vi "Navigate and Wait.vi"(7 "html Source (URL)":bool, 8 "Error In":errorcluster, 9 "Timeout (Inf)":i32=-1, 10 "Source":string, 11 "WebView in":refnum<class "WebView.lvclass">) -> (0 "Error Out":errorcluster, 2 "Timed Out":bool, 3 "WebView out":refnum<class "WebView.lvclass">)   [LabVIEW 2020, in "WebView.lvclass"]
uses:
  WebView.lvclass
  <vilib>/sklein/WebView2/Libs/Microsoft.Web.WebView2.Core.dll
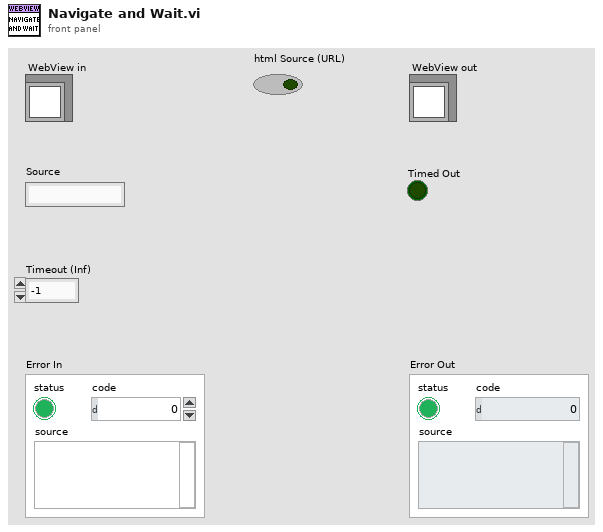
[diagram p1: front panel]
types:
  T1 = typedef "WebView.lvclass/Events--cluster.ctl" = cluster{"Navigation Complete Event":refnum<user-event>, "Source Changed Event":refnum<user-event>, "Document Title Changed Event":refnum<user-event>, "Status Bar Text Changed":refnum<user-event>, "Web Message Received":refnum<user-event>, "Window Close Requested":refnum<user-event>, "DOM Loaded":refnum<user-event>, "Navigation Started Event":refnum<user-event>}
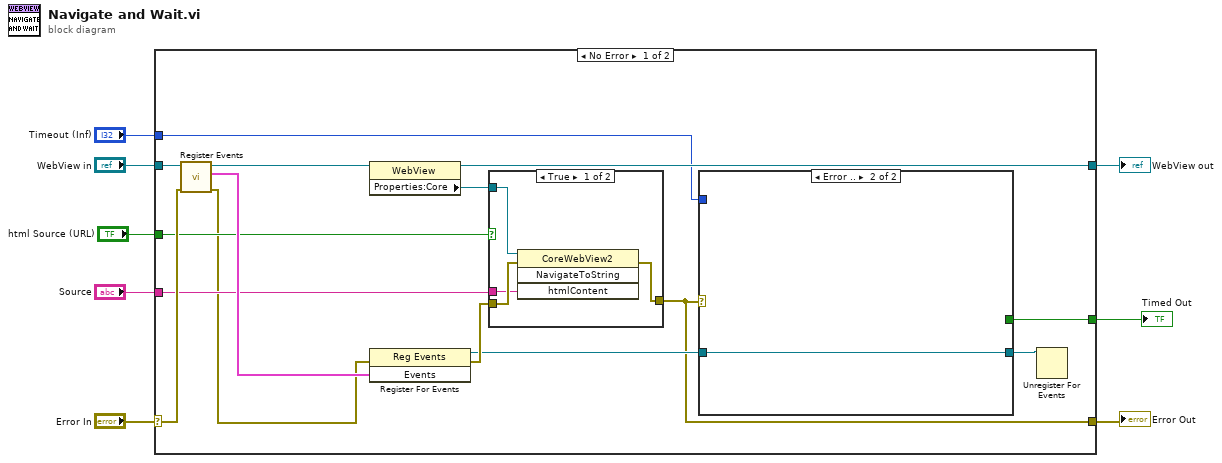
[diagram p0: block diagram]
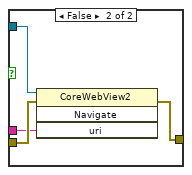
[diagram p2: hidden frame]
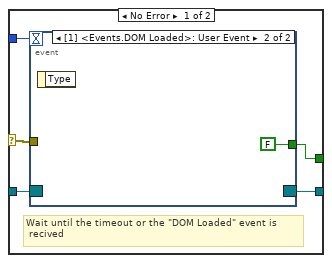
[diagram p3: hidden frame]
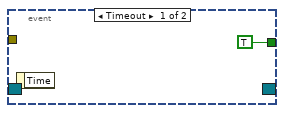
[diagram p4: hidden frame]
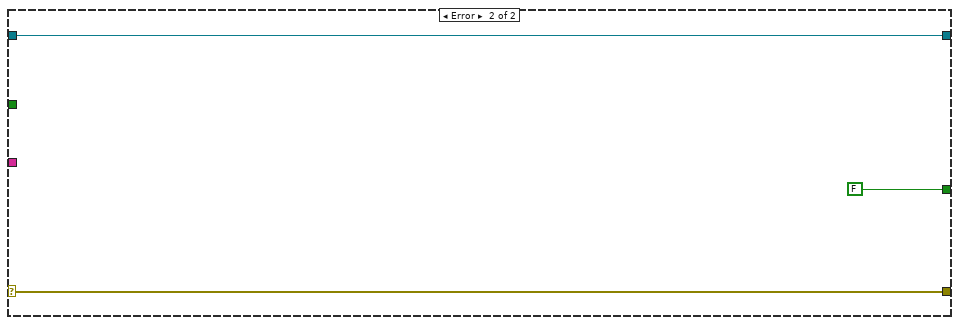
[diagram p5: hidden frame]
diagram:
  n1 = case shown="No Error" "Error In" {
    selector: "Error In" -> [w15 w42]
    tunnel: [w9 w42] -> w7
    tunnel: [w20 w41] -> w5
    tunnel: "WebView in" -> [w18 w41]
    tunnel: [w14 FALSE] -> w4
    tunnel: "Source" -> [w13 _]
    tunnel: "html Source (URL)" -> [w12 _]
    tunnel: "Timeout (Inf)" -> [w11 _]
    frame No Error {
      n2 = call-dynamic "Register Events.vi"("Error In"=w15, "WebView in"=w18) -> ("Error Out"=w10:errorcluster, "Events"=w16:T1, "WebView out"=w17:refnum<class "WebView.lvclass">)  [unwired: 7 in]
      n3 = property class="WebView"(reference=w17) -> (reference out=w20:refnum<class "WebView.lvclass">, "Properties:Core"=w19:refnum<k24>)  [unwired: 1 in, 1 out]
      n4 = register-events(error in=w10, w16) -> (reference out=w22:refnum<event-registration>, error out=w23:errorcluster)  [unwired: 1 in]
      n5 = case shown="True" w12 {
        tunnel: w23 -> [w27 w31]
        tunnel: w13 -> [w26 w30]
        tunnel: [w25 w29] -> w9
        tunnel: w19 -> [w24 w28]
        frame True {
          n6 = invoke class="CoreWebView2" method="NavigateToString"(reference=w24, error in=w27, "htmlContent"=w26) -> (error out=w25:errorcluster)  [unwired: 1 in, 3 out]
        }
        frame False {
          n7 = invoke class="CoreWebView2" method="Navigate"(reference=w28, error in=w31, "uri"=w30) -> (error out=w29:errorcluster)  [unwired: 1 in, 3 out]
        }
      }
      n8 = case shown="Error .." w9 {
        selector: w9 -> [w32 _]
        tunnel: w22 -> [w36 w39]
        tunnel: [w35 _] -> w14
        tunnel: w11 -> [w34 _]
        tunnel: [w33 w39] -> w21
        frame No Error {
          # "Wait until the timeout or the \"DOM Loaded\" event is\n recived"
          n9 = event shown="[1] <Events.DOM Loaded>: User Event" {
            selector: w36 -> [_ _]
            dyn-events: [_ _] -> w33
            timeout: w34 -> [_ _]
            tunnel: [TRUE FALSE] -> w35
            tunnel: w32 -> [_ _]
            event Timeout {
              n10 = event-data() -> ()  [unwired: 1 in, 1 out]
            }
            event User Event {
              n11 = event-data() -> ()  [unwired: 1 in, 1 out]
            }
          }
        }
        frame Error {
        }
      }
      n12 = Unregister For Events(event registration refnum=w21) -> ()  [unwired: 1 in, 1 out]
    }
    frame Error {
    }
  }
  "Error Out" <- w7
  "WebView out" <- w5
  "Timed Out" <- w4
